vi "Set Server State Ref.vi"(10 "Server Internal State Ref":refnum<data-value>, 11 "Template Server in":refnum<class "ctet_mux.lvclass">) -> (3 "Template Server out":refnum<class "ctet_mux.lvclass">)   [LabVIEW 2019, in "ctet_mux.lvlib" / "ctet_mux.lvclass"]
uses:
  ctet_mux.lvclass
  typeDefs/Server State Data.ctl
  ctet_mux.lvclass/ctet_mux.ctl
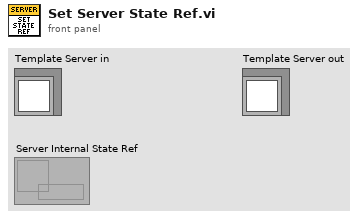
[diagram p1: front panel]
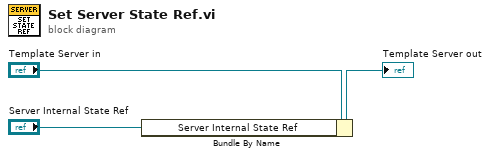
[diagram p0: block diagram]
diagram:
  n1 = Bundle By Name(cluster="Template Server in", "Server Internal State Ref"="Server Internal State Ref") -> (→"Template Server out":refnum<class "ctet_mux.lvclass">)
